vi "Final_v1.vi"() -> ()   [LabVIEW 2019]
uses:
  src/class/mqtt/mqttTypedef/mqttBroker.ctl
  src/class/mqtt/mqttTypedef/mqttConnectionFlags.ctl
  src/class/mqtt/mqttTypedef/mqttWillInformation.ctl
  src/class/mqtt/mqttConfigFunction.ctl
  src/class/mqtt/mqttTXqueue/mqttTXdataQueueFunction.ctl
  src/class/mqtt/mqttTXqueue/mqttRXsubscriptionEventFunction.ctl
  src/class/mqtt/mqtt.lvclass
panel:
  out "error out":errorcluster
  in  "Disconnect":bool
  in  "Connect":bool
  out "MQTT Status":bool
  out "電暖爐":bool
  in  "電暖爐 手動開關":bool
  out "Temp L Flag":bool
  out "Temp H Flag":bool
  in  "Slide":dbl(slide) scale=0.0..40.0
  out "Door Flag":bool
  in  "Boolean":bool
  out "電扇":bool
  out "Boolean 73":bool
  out "Boolean 72":bool
  out "Boolean 71":bool
  out "Boolean 43":bool
  out "Boolean 70":bool
  out "Boolean 69":bool
  out "Boolean 68":bool
  out "Boolean 67":bool
  out "Boolean 66":bool
  out "Boolean 65":bool
  out "Boolean 64":bool
  out "Boolean 63":bool
  out "Boolean 62":bool
  out "Boolean 61":bool
  out "Boolean 60":bool
  out "Boolean 59":bool
  out "Boolean 58":bool
  out "Boolean 57":bool
  out "Boolean 56":bool
  out "Boolean 55":bool
  out "Boolean 54":bool
  out "Boolean 53":bool
  out "Boolean 52":bool
  out "Boolean 51":bool
  out "Boolean 50":bool
  out "Boolean 49":bool
  out "Boolean 48":bool
  out "Boolean 47":bool
  out "Boolean 46":bool
  out "Boolean 45":bool
  out "Boolean 44":bool
  out "Boolean 43":bool
  out "Boolean 42":bool
  out "Boolean 41":bool
  out "Boolean 40":bool
  out "Boolean 39":bool
  out "Boolean 38":bool
  out "Boolean 37":bool
  out "Boolean 36":bool
  out "Boolean 35":bool
  out "Boolean 34":bool
  out "Boolean 33":bool
  out "Boolean 32":bool
  out "Boolean 31":bool
  out "Boolean 30":bool
  out "Boolean 29":bool
  in  "電扇 手動開關":bool
  in  "Color Box":u32(colorbox)
  in  "電燈 手動開關":bool
  out "Table":string[][](table)
  in  "Stop Button":bool
  out "溫度過低":bool
  out "溫度過高":bool
  out "溫度下限(*C)":dbl
  out "溫度上限(*C)":dbl
  in  "溫度上下限":cluster{dbl, dbl}(slide) scale=0.0..40.0
  out "溫度表":dbl(slide) scale=0.0..40.0
  out "溫度(*C)":dbl format="%#.2g"
  out "開門":bool
  out "電燈":bool
  # "MQTT"
  # "溫度計"
  # "監控介面"
  # "現在時間"
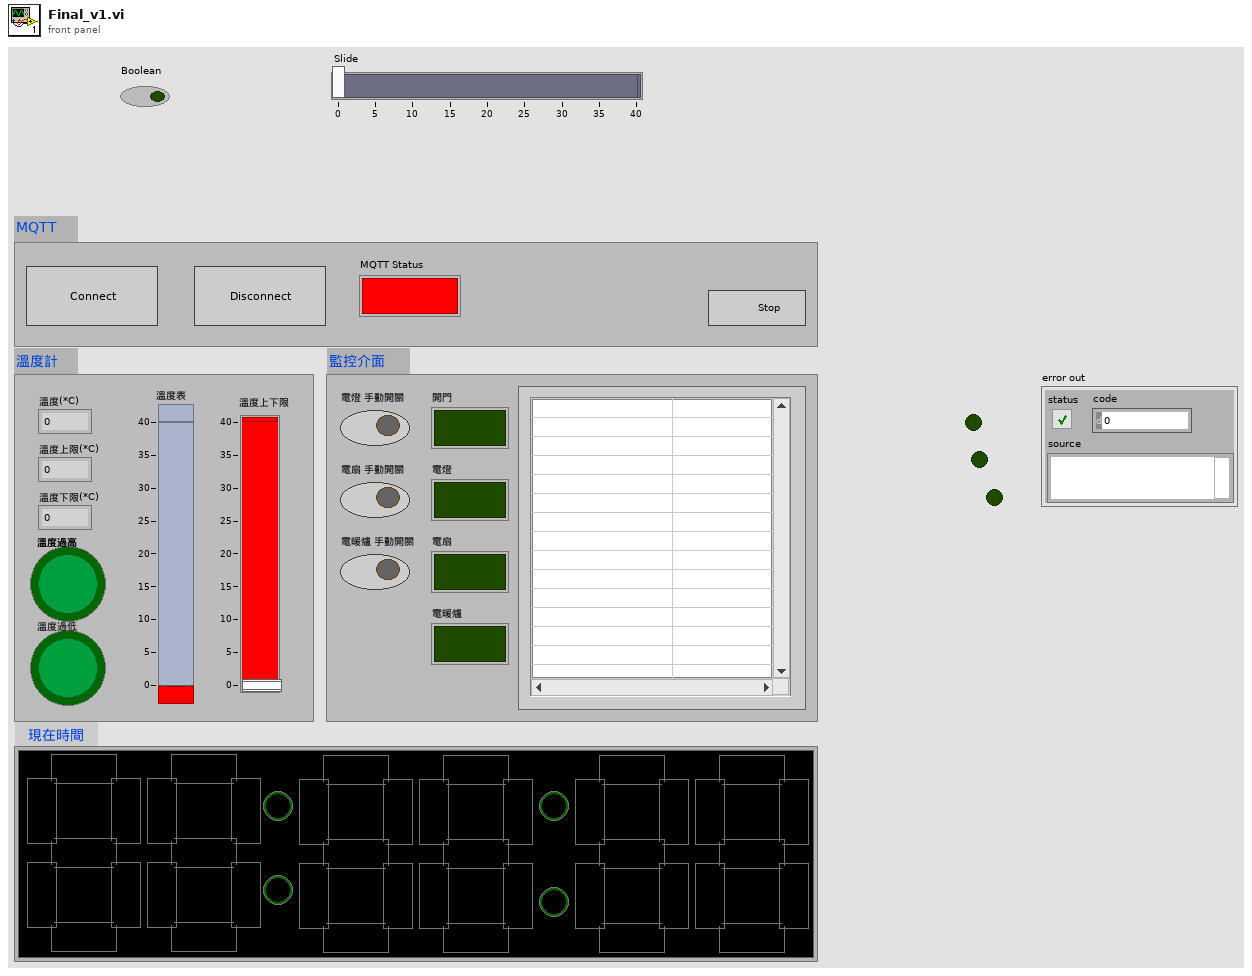
[diagram p1: front panel]
types:
  T1 = typedef "mqttRXsubscriptionEventFunction.ctl" = enum16{"init", "deinit", "getEventRef", "event"}
  T2 = typedef "mqttTXdataQueueFunction.ctl" = enum16{"init", "deinit", "getQueue", "enqueue"}
  T3 = typedef "mqtt.lvclass/mqttConfigFunction.ctl" = enum16{"init", "deinit", "set", "get"}
  T4 = typedef "mqttWillInformation.ctl" = cluster{"User Name":string, "Password":string}
  T5 = typedef "mqttConnectionFlags.ctl" = cluster{"reserved":bool, "clean session":bool, "will flag":bool, "willQOS":enum8{"At most once", "At least once", "Exactly once", "Reserved"}, "will retain":bool, "password":bool, "user name":bool}
  T6 = typedef "mqttBroker.ctl" = cluster{"address":string, "port":u16, "connTimeout":i32, "writeTimeout":i32, "readTimeout":i32, "subTimeout":i32}
  T7 = enum8{"Enabled", "Disabled", "Disabled and Grayed Out"}
  T8 = cluster{bool, bool, bool, bool, bool, bool, bool}[]
  T9 = cluster{bool, bool, bool, bool, bool, bool, bool}
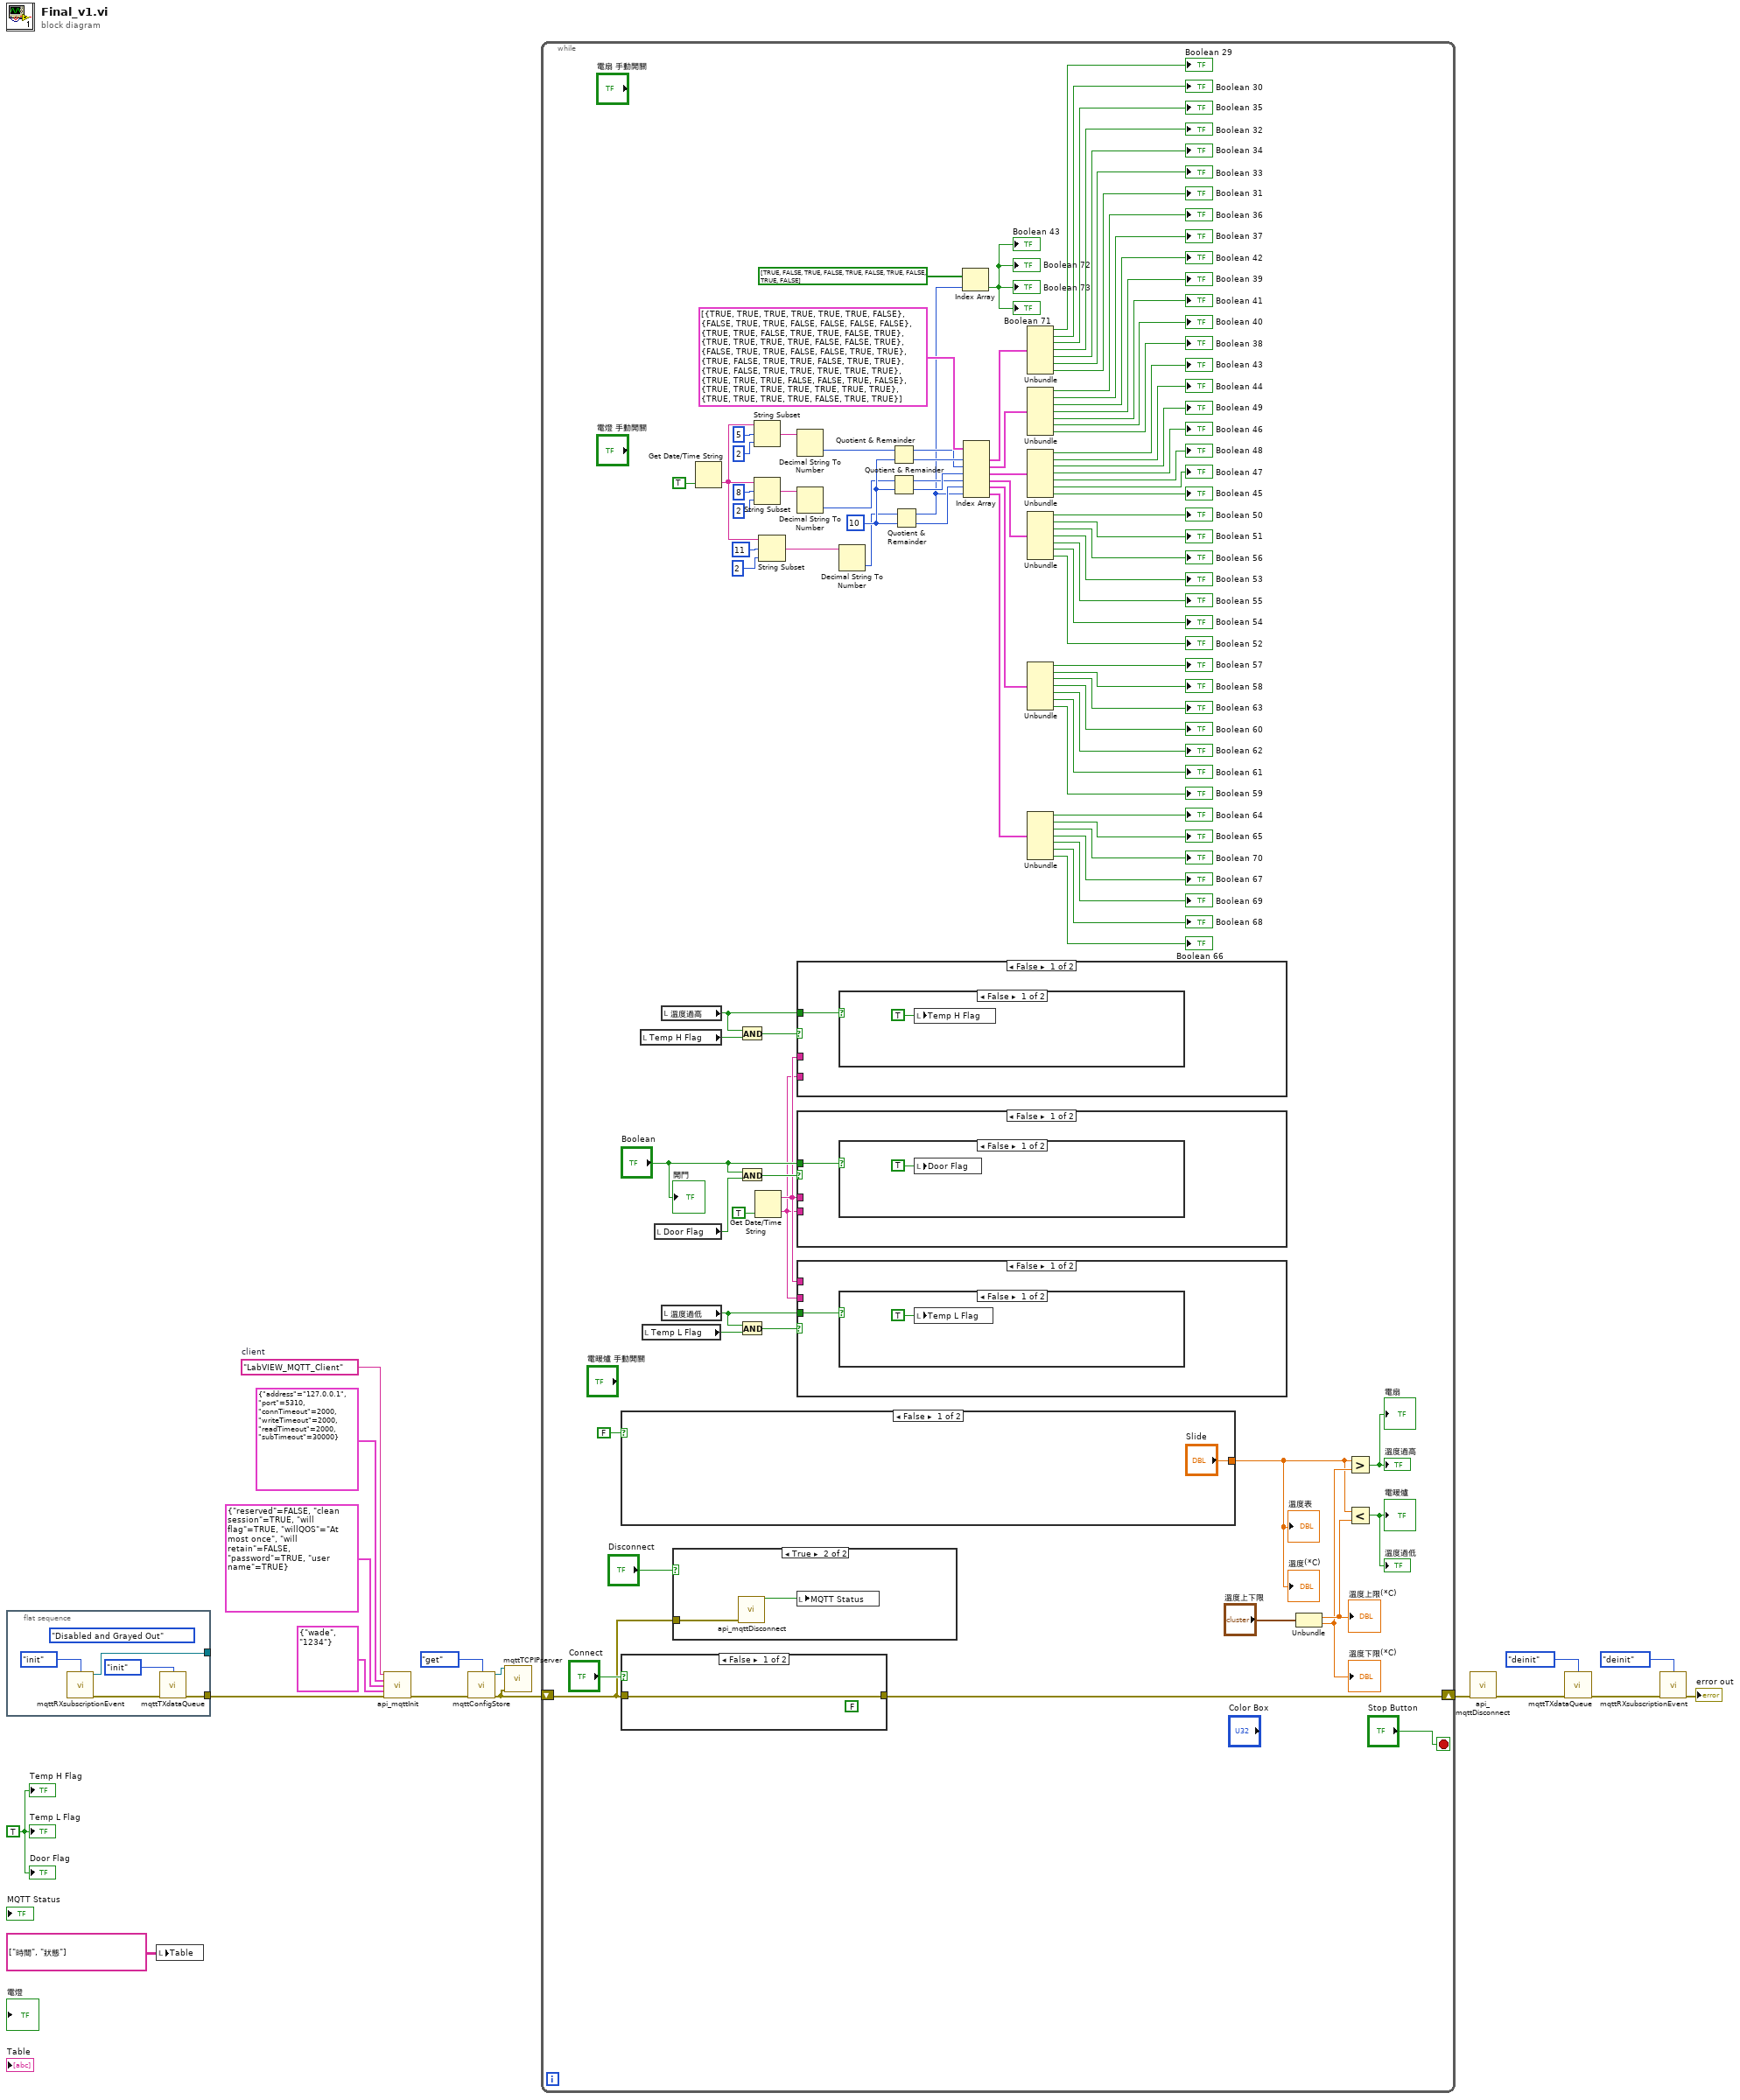
[diagram p0: block diagram]
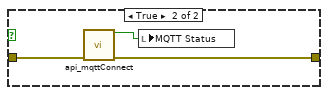
[diagram p3: hidden frame]
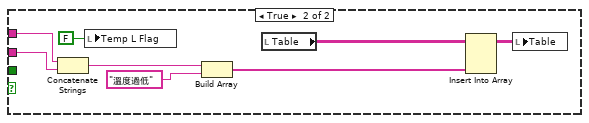
[diagram p5: hidden frame]
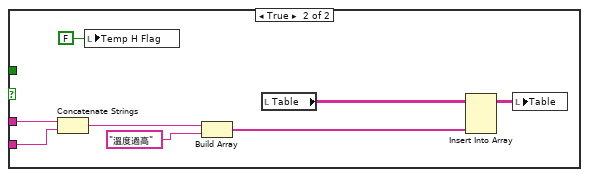
[diagram p7: hidden frame]
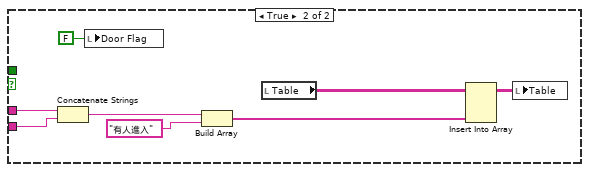
[diagram p9: hidden frame]
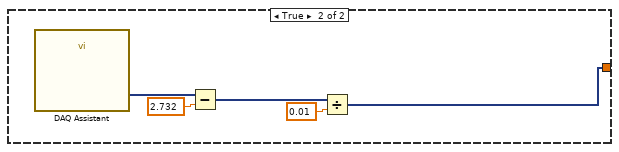
[diagram p10: hidden frame]
diagram:
  w12 = "LabVIEW_MQTT_Client"  # client
  w16 = TRUE ("Door Flag")
  n1 = flat-sequence {
    tunnel: [w21] -> w14
    tunnel: [w18] -> _
    frame #0 {
      (unwired) T7."Disabled and Grayed Out" ("Disabled")
      n2 = call "mqttRXsubscriptionEvent.vi"("function"=mqttRXsubscriptionEventFunction."init") -> ("subscriptionData"=w18:refnum<user-event>, "error out"=w20:errorcluster)  [unwired: 13 in]
      n3 = call "mqttTXdataQueue.vi"("function"=mqttTXdataQueueFunction."init", "error in (no error)"=w20) -> ("error out"=w21:errorcluster)  [unwired: 12 in, 1 out]
    }
  }
  n4 = local write "Table"(string[][] [["時間", "狀態"]]) -> ()
  n5 = call "api_mqttInit.vi"("client"=w12, "broker"=T6 {"address"="127.0.0.1", "port"=5310, "connTimeout"=2000, "writeTimeout"=2000, "readTimeout"=2000, "subTimeout"=30000}, "connFlags"=T5 {"reserved"=FALSE, "clean session"=TRUE, "will flag"=TRUE, "willQOS"=enum."At most once", "will retain"=FALSE, "password"=TRUE, "user name"=TRUE}, "User Info"=T4 {"User Name"="wade", "Password"="1234"}, "error in (no error)"=w14) -> ("error out"=w13:errorcluster)  [unwired: 10 in]
  n6 = call "mqttConfigStore.vi"("function"=mqttConfigFunction."get", "error in (no error)"=w13) -> ("mqtt.lvclass out"=w8:refnum<class "mqtt.lvclass">, "error out"=w2:errorcluster)  [unwired: 12 in]
  n7 = call "mqttTCPIPserver.vi"("mqtt.lvclass"=w8, "error in (no error)"=w2) -> ()  [unwired: 12 in, 2 out]
  n8 = while {
    shift-right: [w24] -> w1
    shift-left: w2 -> [w25]
    stop <- "Stop Button" stop-if-true
    w59 = 10 ("y")
    n9 = case shown="False" FALSE {
      tunnel: ["Slide" w156] -> w37
      frame False {
      }
      frame True {
        n10 = call "DAQ Assistant"() -> ("data"=w157:dynamicdata)  [unwired: 17 in, 2 out]
        n11 = Subtract(x=w157, y=2.732) -> (x-y=w160:dynamicdata)
        n12 = Divide(x=w160, y=0.01) -> (x/y=w156:dynamicdata)
      }
    }
    "溫度(*C)" <- w37
    "溫度表" <- w37
    n13 = case shown="False" "Connect" {
      tunnel: w25 -> [w121 w124]
      tunnel: [w121 w123] -> w24
      frame False {
        (unwired) FALSE ("success")
      }
      frame True {
        n14 = call "api_mqttConnect.vi"("error in (no error)"=w124) -> ("success"=w122:bool, "error out"=w123:errorcluster)  [unwired: 11 in, 2 out]
        n15 = local write "MQTT Status"(w122) -> ()
      }
    }
    n16 = local read "Temp H Flag"() -> (w36:bool)
    n17 = local read "Temp L Flag"() -> (w33:bool)
    n18 = local read "Door Flag"() -> (w40:bool)
    n19 = local read "溫度過高"() -> (w34:bool)
    n20 = local read "溫度過低"() -> (w31:bool)
    n21 = case shown="True" "Disconnect" {
      tunnel: w25 -> [_ w120]
      frame False {
      }
      frame True {
        n22 = call "api_mqttDisconnect.vi"("error in (no error)"=w120) -> ("success"=w119:bool)  [unwired: 13 in, 1 out]
        n23 = local write "MQTT Status"(w119) -> ()
      }
    }
    n24 = Get Date/Time String(want seconds? (F)=TRUE) -> (time string=w50:string)  [unwired: 2 in, 1 out]
    n25 = And(x=w34, y=w36) -> (x .and. y?=w35:bool)
    n26 = And(x="Boolean", y=w40) -> (x .and. y?=w39:bool)
    n27 = And(x=w31, y=w33) -> (x .and. y?=w32:bool)
    n28 = String Subset(string=w50, offset (0)=5, length (rest)=2 ("length (rest)")) -> (substring=w69:string)
    n29 = String Subset(string=w50, offset (0)=8, length (rest)=2 ("length (rest)")) -> (substring=w68:string)
    n30 = Get Date/Time String(want seconds? (F)=TRUE) -> (date string=w30:string, time string=w29:string)  [unwired: 2 in]
    n31 = String Subset(string=w50, offset (0)=11, length (rest)=2 ("length (rest)")) -> (substring=w61:string)
    n32 = Decimal String To Number(string=w69) -> (number=w60:i32)  [unwired: 2 in, 1 out]
    n33 = Decimal String To Number(string=w68) -> (number=w58:i32)  [unwired: 2 in, 1 out]
    n34 = case shown="False" w35 {
      tunnel: w30 -> [_ w139]
      tunnel: w29 -> [_ w138]
      tunnel: w34 -> [w135 _]
      frame False {
        n35 = case shown="False" w135 {
          frame False {
            n36 = local write "Temp H Flag"(TRUE) -> ()
          }
          frame True {
          }
        }
      }
      frame True {
        n37 = Concatenate Strings(w139, w138) -> (w142:string)
        n38 = local write "Temp H Flag"(FALSE ("Temp H Flag")) -> ()
        n39 = Build Array(w142, "溫度過高") -> (w141:string[])
        n40 = local read "Table"() -> (w144:string[][])
        n41 = Insert Into Array(array=w144, new element=w141) -> (w140:string[][])  [unwired: 2 in]
        n42 = local write "Table"(w140) -> ()
      }
    }
    n43 = case shown="False" w39 {
      tunnel: w30 -> [_ w154]
      tunnel: w29 -> [_ w153]
      tunnel: "Boolean" -> [w145 _]
      frame False {
        n44 = case shown="False" w145 {
          frame False {
            n45 = local write "Door Flag"(TRUE ("Door Flag")) -> ()
          }
          frame True {
          }
        }
      }
      frame True {
        n46 = Concatenate Strings(w154, w153) -> (w151:string)
        n47 = local write "Door Flag"(FALSE ("Door Flag")) -> ()
        n48 = Build Array(w151, "有人進入") -> (w150:string[])
        n49 = local read "Table"() -> (w148:string[][])
        n50 = Insert Into Array(array=w148, new element=w150) -> (w147:string[][])  [unwired: 2 in]
        n51 = local write "Table"(w147) -> ()
      }
    }
    n52 = case shown="False" w32 {
      tunnel: w31 -> [w125 _]
      tunnel: w30 -> [_ w133]
      tunnel: w29 -> [_ w132]
      frame False {
        n53 = case shown="False" w125 {
          frame False {
            n54 = local write "Temp L Flag"(TRUE ("Temp L Flag")) -> ()
          }
          frame True {
          }
        }
      }
      frame True {
        n55 = Concatenate Strings(w133, w132) -> (w131:string)
        n56 = local write "Temp L Flag"(FALSE ("Temp L Flag")) -> ()
        n57 = Build Array(w131, "溫度過低") -> (w129:string[])
        n58 = local read "Table"() -> (w128:string[][])
        n59 = Insert Into Array(array=w128, new element=w129) -> (w127:string[][])  [unwired: 2 in]
        n60 = local write "Table"(w127) -> ()
      }
    }
    n61 = Decimal String To Number(string=w61) -> (number=w57:i32)  [unwired: 2 in, 1 out]
    n62 = Quotient & Remainder(x=w60, y=w59) -> (x-y*floor(x/y)=w55:i32, floor(x/y)=w56:i32)
    n63 = Quotient & Remainder(x=w58, y=w59) -> (x-y*floor(x/y)=w53:i32, floor(x/y)=w54:i32)
    n64 = Quotient & Remainder(x=w57, y=w59) -> (x-y*floor(x/y)=w49:i32, floor(x/y)=w52:i32)
    n65 = Index Array(array=bool[] [TRUE, FALSE, TRUE, FALSE, TRUE, FALSE, TRUE, FALSE, TRUE, FALSE], index=w49) -> (element=→"Boolean 43" →"Boolean 71" →"Boolean 72" →"Boolean 73":bool)
    n66 = Index Array(array=T8 [{TRUE, TRUE, TRUE, TRUE, TRUE, TRUE, FALSE}, {FALSE, TRUE, TRUE, FALSE, FALSE, FALSE, FALSE}, {TRUE, TRUE, FALSE, TRUE, TRUE, FALSE, TRUE}, {TRUE, TRUE, TRUE, TRUE, FALSE, FALSE, TRUE}, {FALSE, TRUE, TRUE, FALSE, FALSE, TRUE, TRUE}, {TRUE, FALSE, TRUE, TRUE, FALSE, TRUE, TRUE}, {TRUE, FALSE, TRUE, TRUE, TRUE, TRUE, TRUE}, {TRUE, TRUE, TRUE, FALSE, FALSE, TRUE, FALSE}, {TRUE, TRUE, TRUE, TRUE, TRUE, TRUE, TRUE}, {TRUE, TRUE, TRUE, TRUE, FALSE, TRUE, TRUE}], index #1=w56, index #2=w55, index #3=w54, index #4=w53, index #5=w52, index #6=w49) -> (element #1=w117:T9, element #2=w116:T9, element #3=w115:T9, element #4=w114:T9, element #5=w113:T9, element #6=w112:T9)
    n67 = Unbundle(w117) -> (→"Boolean 29":bool, →"Boolean 30":bool, →"Boolean 35":bool, →"Boolean 32":bool, →"Boolean 34":bool, →"Boolean 33":bool, →"Boolean 31":bool)
    n68 = Unbundle(w116) -> (→"Boolean 36":bool, →"Boolean 37":bool, →"Boolean 42":bool, →"Boolean 39":bool, →"Boolean 41":bool, →"Boolean 40":bool, →"Boolean 38":bool)
    n69 = Unbundle(w115) -> (→"Boolean 43":bool, →"Boolean 44":bool, →"Boolean 49":bool, →"Boolean 46":bool, →"Boolean 48":bool, →"Boolean 47":bool, →"Boolean 45":bool)
    n70 = Unbundle(w114) -> (→"Boolean 50":bool, →"Boolean 51":bool, →"Boolean 56":bool, →"Boolean 53":bool, →"Boolean 55":bool, →"Boolean 54":bool, →"Boolean 52":bool)
    n71 = Unbundle(w113) -> (→"Boolean 57":bool, →"Boolean 58":bool, →"Boolean 63":bool, →"Boolean 60":bool, →"Boolean 62":bool, →"Boolean 61":bool, →"Boolean 59":bool)
    n72 = Unbundle(w112) -> (→"Boolean 64":bool, →"Boolean 65":bool, →"Boolean 70":bool, →"Boolean 67":bool, →"Boolean 69":bool, →"Boolean 68":bool, →"Boolean 66":bool)
    n73 = Unbundle("溫度上下限") -> (w45:dbl, w44:dbl)
    "溫度上限(*C)" <- w45
    "溫度下限(*C)" <- w44
    n74 = Greater?(x=w37, y=w44) -> (0:→"溫度過高" →"電扇":bool)
    n75 = Less?(x=w37, y=w45) -> (x < y?=→"溫度過低" →"電暖爐":bool)
    "開門" <- "Boolean"
  }
  n76 = call "api_mqttDisconnect.vi"("error in (no error)"=w1) -> ("error out"=w6:errorcluster)  [unwired: 13 in, 1 out]
  n77 = call "mqttTXdataQueue.vi"("function"=mqttTXdataQueueFunction."deinit", "error in (no error)"=w6) -> ("error out"=w4:errorcluster)  [unwired: 12 in, 1 out]
  n78 = call "mqttRXsubscriptionEvent.vi"("function"=mqttRXsubscriptionEventFunction."deinit", "error in (no error)"=w4) -> ("error out"=→"error out":errorcluster)  [unwired: 12 in, 1 out]
  "Door Flag" <- w16
  "Temp H Flag" <- w16
  "Temp L Flag" <- w16
